vi "Messungaufnehmen.vi"() -> ()   [LabVIEW 2016]
uses:
  <vilib>/Waveform/WDTFileIO.llb/Export Waveform To Spreadsheet File.vi
panel:
  out "HardwareAntwort":string
  out "Waveform Data":waveform(dbl)(graph)
  in  "Timeout (10000)":u32=10000
  out "error out":errorcluster
  out "VISA resource name out":refnum<visa-resource-name>
  in  "error in (no error)":errorcluster
  in  "VISA resource name":refnum<visa-resource-name>
  in  "Source Channel (0: Channel 1)":i32(ring) items=["Channel 1"=0, "Channel 2"=1, "Channel 3"=2, "Channel 4"=3, "Waveform Memory 1"=5, "Waveform Memory 2"=6, "Serial Bus 1"=7, "Serial Bus 2"=8, "Digital Bus Low"=9, "Digital Bus High "=10, "Digital Bus 1"=11, "Digital Bus 2"=12, "Function 1"=32, "Function 2"=33, "Function 3"=34, "Function 4"=35, "Math 1"=36, "Math 2"=37, "Math 3"=38, "Math 4"=39]
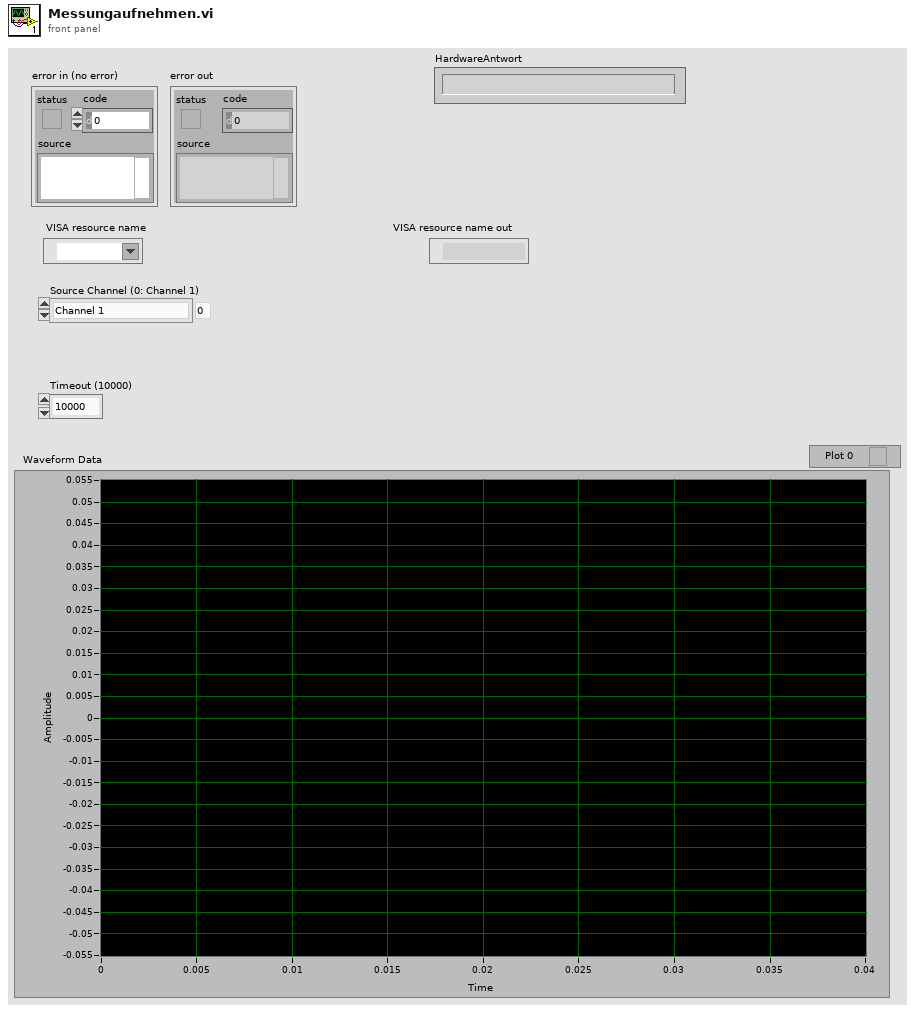
[diagram p1: front panel]
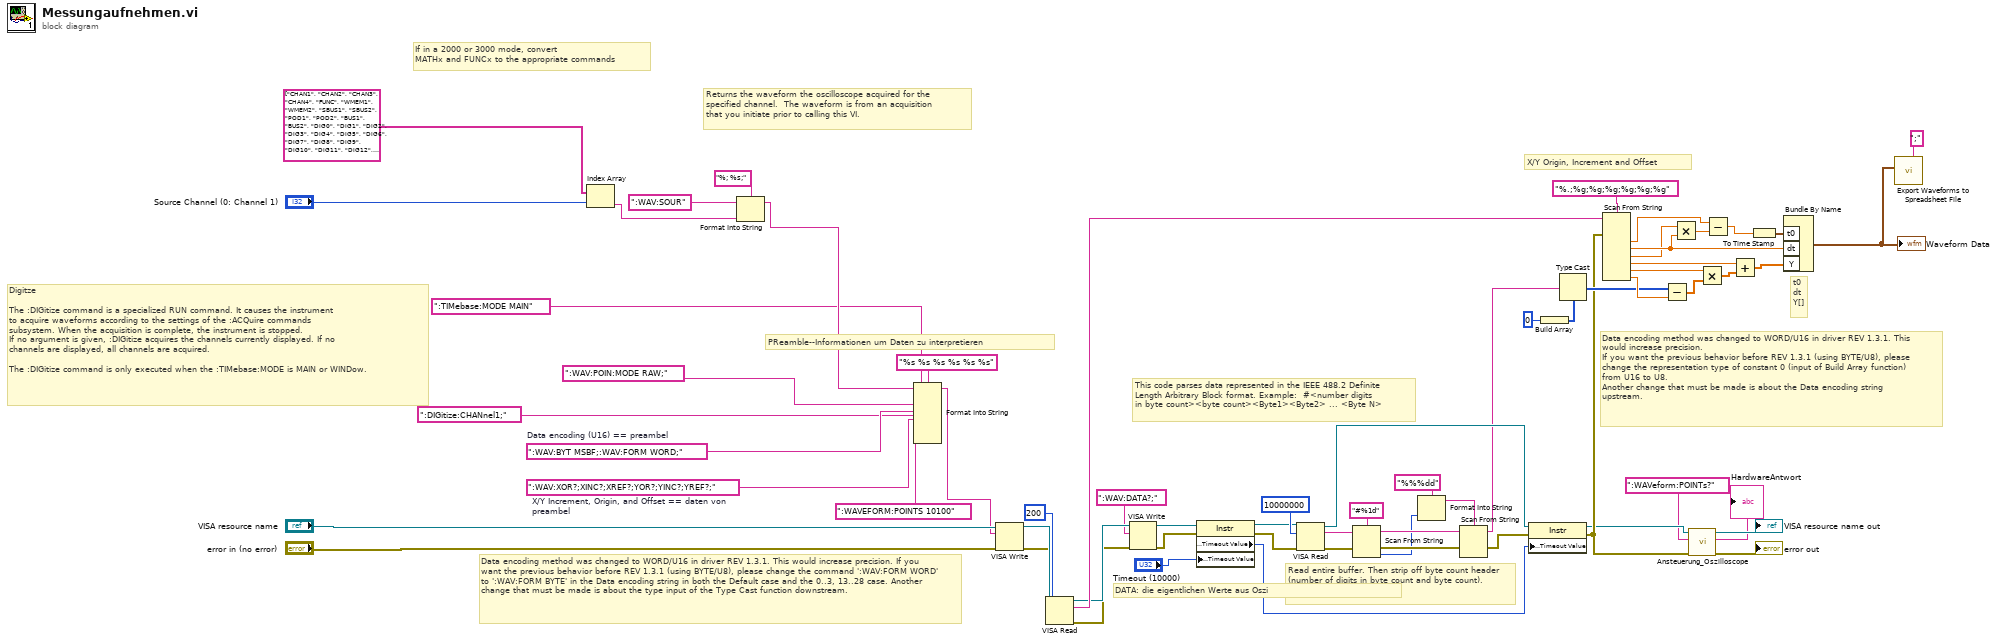
[diagram p0: block diagram]
diagram:
  w19 = ":WAV:XOR?;XINC?;XREF?;YOR?;YINC?;YREF?;"  # X/Y Increment, Origin, and Offset == daten von preambel
  w20 = ":WAV:BYT MSBF;:WAV:FORM WORD;"  # Data encoding (U16) == preambel
  # "DATA: die eigentlichen Werte aus Oszi"
  # "Digitze\n\nThe :DIGitize command is a specialized RUN command. It causes the instrument\nto acquire waveforms according to the settings of the :ACQuire commands\nsubsystem. When the acquisition is complete, the instrument is stopped.\nIf no argument is given, :DIGitize acquires the channels currently displayed. If no\nchannels are displayed, all channels are acquired.\n\nThe :DIGitize command is only executed when the :TIMebase:MODE is MAIN or WINDow."
  # "PReamble--Informationen um Daten zu interpretieren"
  # "Data encoding method was changed to WORD/U16 in driver REV 1.3.1. This would increase precision. If you want the previous behavior before REV 1.3.1 (using BYTE/U8), please change the command ':WAV:FORM WORD' to ':WAV:FORM BYTE' in the Data encoding string in both the Default case and the 0..3, 13..28 case. Another change that must be made is about the type input of the Type Cast function downstream."
  # "Data encoding method was changed to WORD/U16 in driver REV 1.3.1. This would increase precision. \nIf you want the previous behavior before REV 1.3.1 (using BYTE/U8), please change the representation type of constant 0 (input of Build Array function) from U16 to U8. \nAnother change that must be made is about the Data encoding string upstream."
  # "If in a 2000 or 3000 mode, convert\nMATHx and FUNCx to the appropriate commands"
  # "Read entire buffer. Then strip off byte count header (number of digits in byte count and byte count)."
  # "This code parses data represented in the IEEE 488.2 Definite \nLength Arbitrary Block format. Example:  #<number digits \nin byte count><byte count><Byte1><Byte2> ... <Byte N>"
  # "t0\ndt\nY[]"
  # "X/Y Origin, Increment and Offset"
  # "Returns the waveform the oscilloscope acquired for the \nspecified channel.  The waveform is from an acquisition \nthat you initiate prior to calling this VI."
  n1 = Index Array(array=string[] ["CHAN1", "CHAN2", "CHAN3", "CHAN4", "FUNC", "WMEM1", "WMEM2", "SBUS1", "SBUS2", "POD1", "POD2", "BUS1", "BUS2", "DIG0", "DIG1", "DIG2", "DIG3", "DIG4", "DIG5", "DIG6", "DIG7", "DIG8", "DIG9", "DIG10", "DIG11", "DIG12", "DIG13", "DIG14", "DIG15", "EXT", "LINE", "WGEN", "FUNC1", "FUNC2", "FUNC3", "FUNC4", "MATH1", "MATH2", "MATH3", "MATH4"], index="Source Channel (0: Channel 1)") -> (element=w12:string)
  n2 = Format Into String(format string="%; %s;", initial string=":WAV:SOUR" ("Eingangs-String"), w12) -> (resulting string=w15:string)  [unwired: 1 in, 1 out]
  n3 = Format Into String(format string="%s %s %s %s %s %s", initial string=w15, ":WAV:POIN:MODE RAW;", w20, w19, ":WAVEFORM:POINTS 10100" ("Eingang 4"), ":DIGitize:CHANnel1;", ":TIMebase:MODE MAIN") -> (resulting string=w16:string)  [unwired: 1 in, 1 out]
  n4 = VISA Write(VISA resource name="VISA resource name", write buffer=w16, error in (no error)="error in (no error)") -> (VISA resource name out=w26:refnum<visa-resource-name>, error out=w25:errorcluster)  [unwired: 1 out]
  n5 = VISA Read(VISA resource name=w26, byte count=u32 200, error in (no error)=w25) -> (VISA resource name out=w45:refnum<visa-resource-name>, read buffer=w63:string, error out=w44:errorcluster)  [unwired: 1 out]
  n6 = VISA Write(VISA resource name=w45, write buffer=":WAV:DATA?;", error in (no error)=w44) -> (VISA resource name out=w46:refnum<visa-resource-name>, error out=w47:errorcluster)  [unwired: 1 out]
  n7 = property class="Instr"(reference=w46, error in=w47, "General Settings:Timeout Value"="Timeout (10000)") -> (reference out=w41:refnum<visa-resource-name>, error out=w40:errorcluster, "General Settings:Timeout Value"=w43:u32)
  n8 = VISA Read(VISA resource name=w41, byte count=u32 10000000, error in (no error)=w40) -> (VISA resource name out=w39:refnum<visa-resource-name>, read buffer=w50:string, error out=w48:errorcluster)  [unwired: 1 out]
  n9 = Scan From String(format string="#%1d", input string=w50, error in=w48) -> (remaining string=w54:string, error out=w52:errorcluster, output 1=w51:i32)  [unwired: 1 in, 2 out]
  n10 = Format Into String(format string="%%%dd", w51) -> (resulting string=w53:string)  [unwired: 2 in, 1 out]
  n11 = Scan From String(format string=w53, input string=w54, error in=w52) -> (remaining string=w36:string, error out=w35:errorcluster)  [unwired: 1 in, 3 out]
  n12 = property class="Instr"(reference=w39, error in=w35, "General Settings:Timeout Value"=w43) -> (reference out=w8:refnum<visa-resource-name>, error out=w9:errorcluster)
  n13 = Build Array(u16 0) -> (w38:u16[])
  n14 = Type Cast(type=w38, x=w36) -> (*(type *) &x=w32:u16[])
  n15 = Scan From String(format string="%.;%g;%g;%g;%g;%g;%g", input string=w63, error in=w9) -> (output 1=w57:dbl, output 2=w61:dbl, output 3=w60:dbl, output 4=w29:dbl, output 5=w31:dbl, output 6=w33:dbl)  [unwired: 1 in, 9 out]
  n16 = Subtract(x=w32, y=w33) -> (x-y=w30:dbl[])
  n17 = Multiply(x=w60, y=w61) -> (x*y=w58:dbl)
  n18 = call "Ansteuerung_Oszilloscope.vi"("Error_in"=w9, "Eingangs-String"=":WAVeform:POINTs?" ("format string"), "VISA-Ressourcenname (optional)"=w8) -> ("Error_out"=→"error out":errorcluster, "HardwareAntwort"=→"HardwareAntwort":string, "VISA-Ressourcenname out (optional)"=→"VISA resource name out":refnum<visa-resource-name>)  [unwired: 6 in]
  n19 = Multiply(x=w31, y=w30) -> (x*y=w28:dbl[])
  n20 = Subtract(x=w57, y=w58) -> (x-y=w59:dbl)
  n21 = Add(x=w29, y=w28) -> (x+y=w27:dbl[])
  n22 = To Time Stamp(1:w59) -> (0:w62:timestamp)
  n23 = Bundle By Name("t0"=w62, "dt"=w61, "Y"=w27) -> (w4:waveform(dbl))  [unwired: 1 out]
  "Waveform Data" <- w4
  n24 = call-poly <vilib>:"Export Waveforms to Spreadsheet File.vi"("delimiter (Tab)"=";", "waveform"=w4) -> ()  [unwired: 8 in, 2 out]
